vi "TangoAttributeChangeAndPeriodicEventTest.vi"() -> ()   [LabVIEW 2013, in "examples.lvlib"]
uses:
  examples.lvlib
  vis/lv-2013/tango_vi.llb/tango.lvlib
  vis/lv-2013/tango_vi.llb/avToDoubleScalar.vi
  vis/lv-2013/tango_vi.llb/avToLongScalar.vi
  vis/lv-2013/tango_vi.llb/avToULongSpectrum.vi
  vis/lv-2013/tango_vi.llb/avToUShortSpectrum.vi
  vis/lv-2013/tango_vi.llb/_TangoSubscribeAttributePeriodicEvent.vi
  vis/lv-2013/tango_vi.llb/_TangoSubscribeAttributeChangeEvent.vi
panel:
  out "Intensity Graph":u32[][](graph)
  out "Waveform Graph":u16[](graph)
  in  "events types":T1(array[ring])=[enum."PERIODIC_EVENT", enum."PERIODIC_EVENT"]
  in  "events sources":string[][](array[string])=[["sys/tg_test/1", "ushort_spectrum_ro"], ["sys/tg_test/1", "ulong_image_ro"]]
  out "Event Timeout":bool
  in  "timeout (ms)":i32=1000
  out "?":dbl(graph)=-95.9004706383706
  in  "Attribute name":string="long_scalar"
  out "?":i32(graph)=203
  out "Attribute Value":i32
  out "Event Timeout":bool
  in  "timeout (ms)":i32=1000
  in  "?":bool
  out "Attribute Value":dbl
  in  "Device Name":string="sys/tg_test/1"
  in  "Attribute Name":string="double_scalar"
  # "TANGO \"ATTRIBUTE EVENTS\" DEMO"
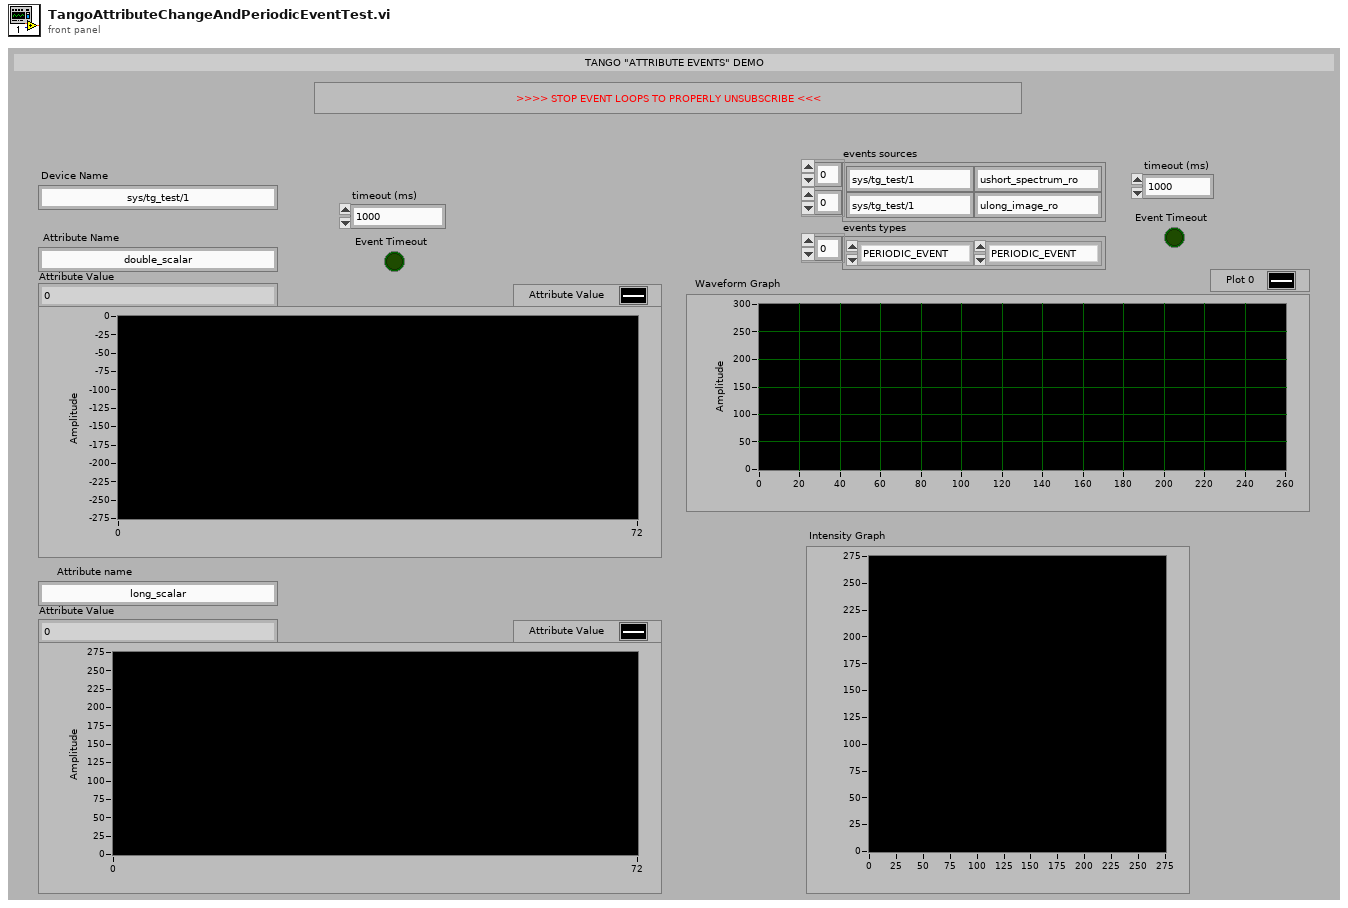
[diagram p1: front panel]
types:
  T1 = enum32{"CHANGE_EVENT", "DEPRECATED_QUALITY_EVENT", "PERIODIC_EVENT", "ARCHIVE_EVENT", "USER_EVENT", "ATTRIBUTE_CONF_EVENT", "DATA_READY_EVENT", "INTERFACE_CHANGE_EVENT", "UNKNOWN_EVENT"}[]
  T2 = cluster{"user event ref":refnum<user-event>, "user event reg refnum":refnum<event-registration>}
  T3 = cluster{"device name":string, "attribute name":string, "quality value":i16, "quality string":string, "timestamp":dbl, "dim. x":i32, "dim. y":i32, "value":u8[], "error code":i32, "error stack":string[], "data type":u16}
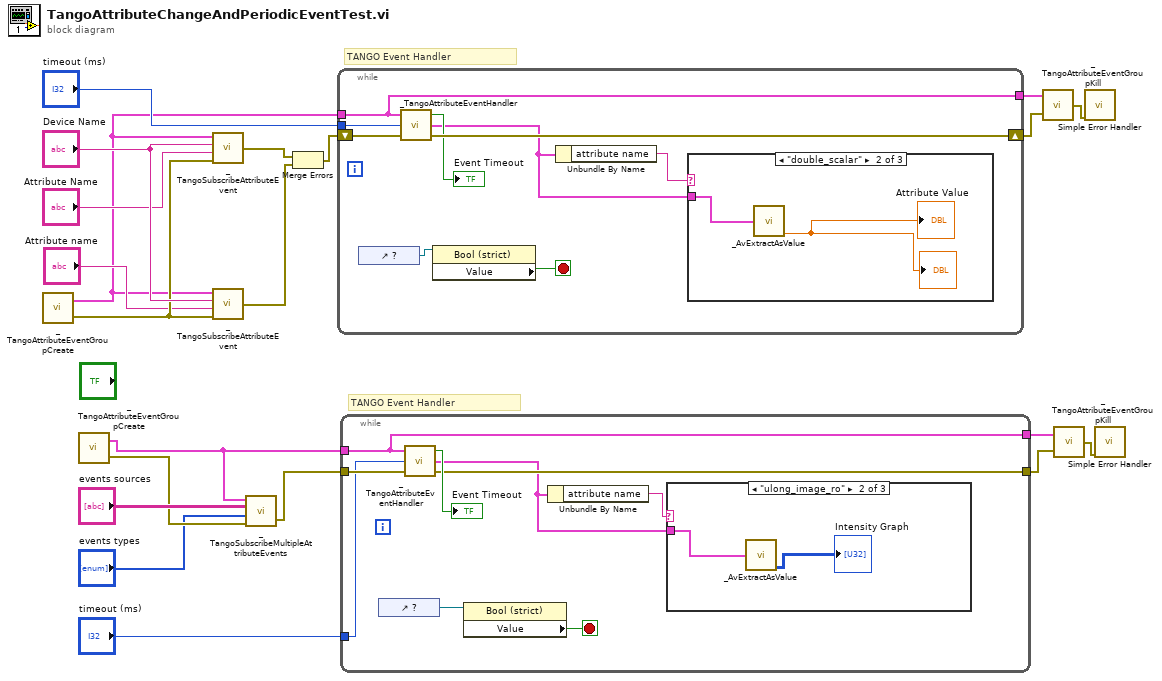
[diagram p0: block diagram]
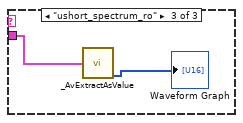
[diagram p3: hidden frame]
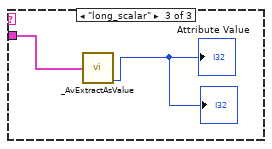
[diagram p5: hidden frame]
diagram:
  # "TANGO Event Handler"
  # "TANGO Event Handler"
  n1 = call "_TangoAttributeEventGroupCreate.vi"() -> ("attribute event ref."=w6:T2, "error out"=w14:errorcluster)  [unwired: 1 in]
  n2 = call "_TangoAttributeEventGroupCreate.vi"() -> ("attribute event ref."=w1:T2, "error out"=w12:errorcluster)  [unwired: 1 in]
  n3 = call-poly "_TangoSubscribeAttributeEvent.vi"("error in"=w14, "attribute name"="Attribute Name", "device name"="Device Name", "attribute event ref."=w6) -> ("error out"=w17:errorcluster)
  n4 = call-poly "_TangoSubscribeAttributeEvent.vi"("error in"=w14, "attribute name"="Attribute name", "device name"="Device Name", "attribute event ref."=w6) -> ("error out"=w16:errorcluster)
  n5 = call "_TangoSubscribeMultipleAttributeEvents.vi"("error in"=w12, "events types"="events types", "events sources"="events sources", "attribute event ref."=w1) -> ("error out"=w10:errorcluster)  [unwired: 1 out]
  n6 = Merge Errors(w17, w16) -> (w15:errorcluster)
  n7 = while {
    shift-right: [w28] -> w4
    shift-left: w15 -> [w25]
    tunnel: "timeout (ms)" -> [w26]
    tunnel: w6 -> [w22]
    tunnel: [w22] -> w5
    stop <- w29 stop-if-true
    n8 = control-ref of="?"() -> (w30:refnum<vi>)
    n9 = call "_TangoAttributeEventHandler.vi"("error in"=w25, "timeout (ms)"=w26, "attribute event ref."=w22) -> ("error out"=w28:errorcluster, "attribute raw data"=w23:T3, "event timeout"=→"Event Timeout":bool)
    n10 = property class="Bool (strict)"(reference=w30) -> ("Value"=w29:bool)  [unwired: 1 in, 2 out]
    n11 = Unbundle By Name(w23) -> ("attribute name"=w27:string)
    n12 = case shown="\"double_scalar\"" w27 {
      tunnel: w23 -> [_ w31 w34]
      frame Default {
      }
      frame "double_scalar" {
        n13 = call-poly "_AvExtractAsValue.vi"("attribute value"=w31) -> ("value"=→"Attribute Value" →"?":dbl)  [unwired: 4 out]
      }
      frame "long_scalar" {
        n14 = call-poly "_AvExtractAsValue.vi"("attribute value"=w34) -> ("value"=→"Attribute Value" →"?":i32)  [unwired: 4 out]
      }
    }
  }
  n15 = while {
    tunnel: w10 -> [w42]
    tunnel: [w40] -> w2
    tunnel: "timeout (ms)" -> [w39]
    tunnel: w1 -> [w36]
    tunnel: [w36] -> w3
    stop <- w43 stop-if-true
    n16 = control-ref of="?"() -> (w35:refnum<vi>)
    n17 = call "_TangoAttributeEventHandler.vi"("error in"=w42, "timeout (ms)"=w39, "attribute event ref."=w36) -> ("error out"=w40:errorcluster, "attribute raw data"=w37:T3, "event timeout"=→"Event Timeout":bool)
    n18 = property class="Bool (strict)"(reference=w35) -> ("Value"=w43:bool)  [unwired: 1 in, 2 out]
    n19 = Unbundle By Name(w37) -> ("attribute name"=w38:string)
    n20 = case shown="\"ulong_image_ro\"" w38 {
      tunnel: w37 -> [_ w45 w46]
      frame Default {
      }
      frame "ulong_image_ro" {
        n21 = call-poly "_AvExtractAsValue.vi"("attribute value"=w45) -> ("value"=→"Intensity Graph":u32[][])  [unwired: 4 out]
      }
      frame "ushort_spectrum_ro" {
        n22 = call-poly "_AvExtractAsValue.vi"("attribute value"=w46) -> ("value"=→"Waveform Graph":u16[])  [unwired: 4 out]
      }
    }
  }
  n23 = call "_TangoAttributeEventGroupKill.vi"("error in"=w4, "attribute event ref."=w5) -> ("error out"=w18:errorcluster)
  n24 = call "_TangoAttributeEventGroupKill.vi"("error in"=w2, "attribute event ref."=w3) -> ("error out"=w9:errorcluster)
  n25 = call <vilib>:"Simple Error Handler.vi"("error in (no error)"=w18) -> ()  [unwired: 4 in, 5 out]
  n26 = call <vilib>:"Simple Error Handler.vi"("error in (no error)"=w9) -> ()  [unwired: 4 in, 5 out]
